vi "FRCts20_WebMethods_ReadData_eventsGet.vi"(8 "error in (no error)":errorcluster, 10 "Single Event":T1, 11 "httpRequestID":u32) -> (0 "error out":errorcluster, 2 "Single Event out":T1, 3 "httpRequestID out":u32)   [LabVIEW 2013]
uses:
  <vilib>/wsapi/NI_WebServices.lvlib
  Web Method Public Interface/FRCts20_WebMethods_ctl_teamIdentifier.ctl
  FRCts20_WebMethods.lvlib
  Web Method Public Interface/FRCts20_WebMethods_ctl_singleEvent.ctl
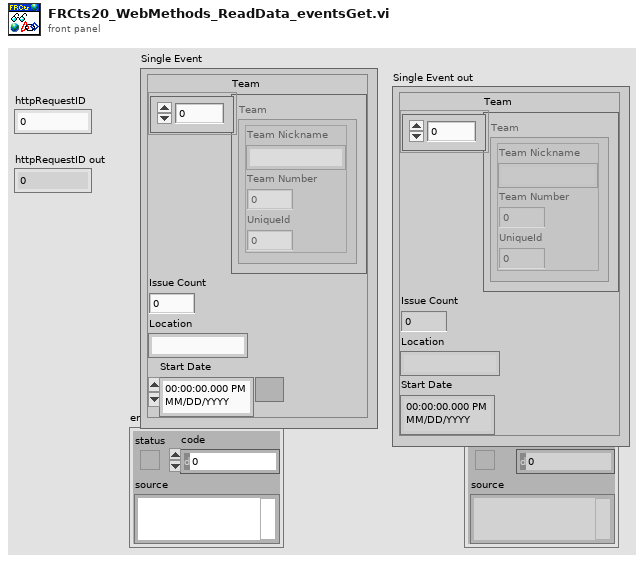
[diagram p1: front panel]
types:
  T1 = typedef "FRCts20_WebMethods.lvlib/FRCts20_WebMethods_ctl_singleEvent.ctl" = cluster{"Team":T2[], "Issue Count":i32, "Location":string, "Start Date ":timestamp}
  T2 = typedef "FRCts20_WebMethods.lvlib/FRCts20_WebMethods_ctl_teamIdentifier.ctl" = cluster{"Team Nickname":string, "Team Number ":u32, "UniqueId":u32}
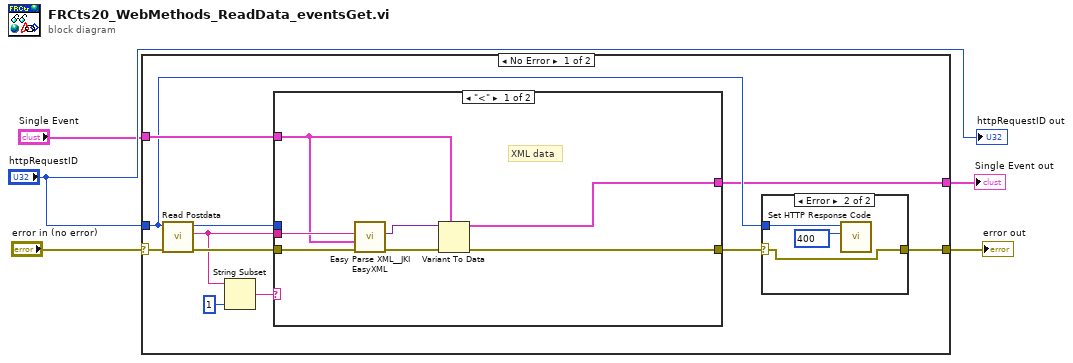
[diagram p0: block diagram]
diagram:
  n1 = case shown="No Error" "error in (no error)" {
    selector: "error in (no error)" -> [w16 w31]
    tunnel: "httpRequestID" -> [w7 _]
    tunnel: "Single Event" -> [w10 w30]
    tunnel: [w8 w31] -> w4
    tunnel: [w6 w30] -> w1
    frame No Error {
      n2 = call <vilib>:"Read Postdata.vi"("error in (no error)"=w16, "httpRequestID"=w7) -> ("error out"=w13:errorcluster, "postdata"=w11:string, "httpRequestID out"=w12:u32)  [unwired: 7 in]
      n3 = String Subset(string=w11, length (rest)=1 ("length (rest)")) -> (substring=w14:string)  [unwired: 1 in]
      n4 = case shown="\"<\"" w14 {
        tunnel: w13 -> [w27 w28]
        tunnel: w12 -> [_ _]
        tunnel: w11 -> [w26 _]
        tunnel: w10 -> [w23 w29]
        tunnel: [w21 w28] -> w9
        tunnel: [w22 w29] -> w6
        frame "<" {
          # "XML data"
          n5 = call <vilib>:"Easy Parse XML__JKI EasyXML.vi"("error in (no error)"=w27, "LabVIEW Data (Type)"=w23, "XML String"=w26) -> ("error out"=w25:errorcluster, "LabVIEW Data"=w24:variant)  [unwired: 7 in]
          n6 = Variant To Data(error in=w25, type=w23, Variant=w24) -> (data=w22:T1, error out=w21:errorcluster)
        }
        frame Default {
        }
      }
      n7 = case shown="Error" w9 {
        selector: w9 -> [w17 w18]
        tunnel: [w17 w18] -> w8
        tunnel: w7 -> [_ w20]
        frame No Error {
        }
        frame Error {
          w19 = 400 items=["100"=100, "101"=101, "200"=200, "201"=201, "202"=202, "203"=203, "204"=204, "205"=205, "206"=206, "300"=300, "301"=301, "302"=302, "303"=303, "304"=304, "305"=305, "306"=306, "307"=307, "400"=400, "401"=401, "402"=402, "403"=403, "404"=404, "405"=405, "406"=406, "407"=407, "408"=408, "409"=409, "410"=410, "411"=411, "412"=412, "413"=413, "414"=414, "415"=415, "416"=416, "417"=417, "500"=500, "501"=501, "502"=502, "503"=503, "504"=504, "505"=505] ("response code (200)")
          n8 = call <vilib>:"Set HTTP Response Code.vi"("response code (200)"=w19, "httpRequestID"=w20) -> ()  [unwired: 8 in, 2 out]
        }
      }
    }
    frame Error {
    }
  }
  "error out" <- w4
  "Single Event out" <- w1
  "httpRequestID out" <- "httpRequestID"
